vi "security system for building (2).vi"() -> ()   [LabVIEW 2020]
panel:
  out "Normal":bool
  out "Fire":bool
  in  "Temp":dbl
  in  "stop":bool
  out "Hot":bool
  out "Cold":bool
  in  "Switch":bool
  in  "Motion sensor":bool
  out "Light":bool
  in  "Stop Time":timestamp
  in  "Start Time":timestamp
  in  "ON/OFF":bool
  out "Normal Alarm":bool
  out "Smoke Alarm":bool
  out "Fire Alarm":bool
  in  "SMOKE LEVEL  SET POINT":dbl(knob) scale=0.0..100.0
  in  "SMOKE   DETECTOR":dbl(knob) scale=0.0..100.0
  in  "TEMP SET POINT":dbl(slide) scale=0.0..100.0
  in  "TEMPERATURE  DETECTOR":dbl(slide) scale=0.0..100.0
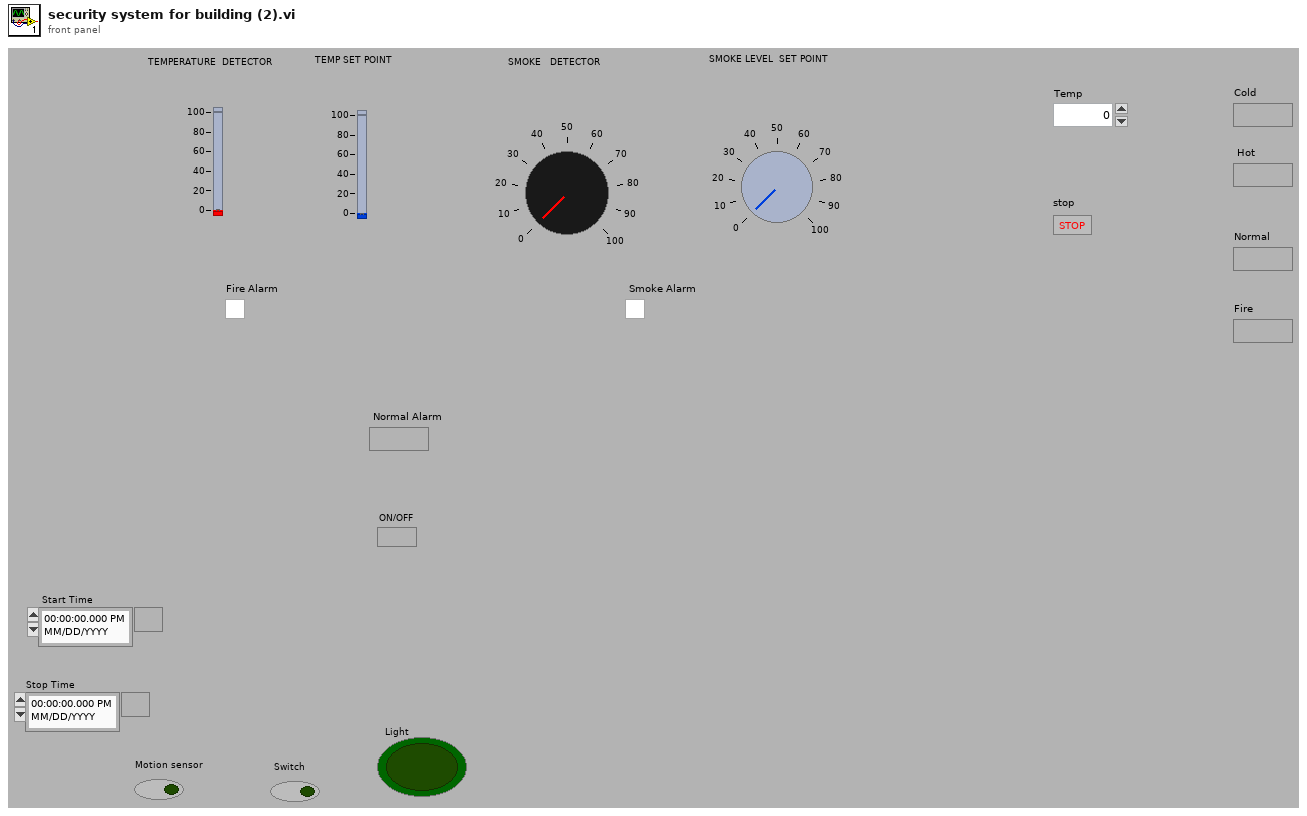
[diagram p1: front panel]
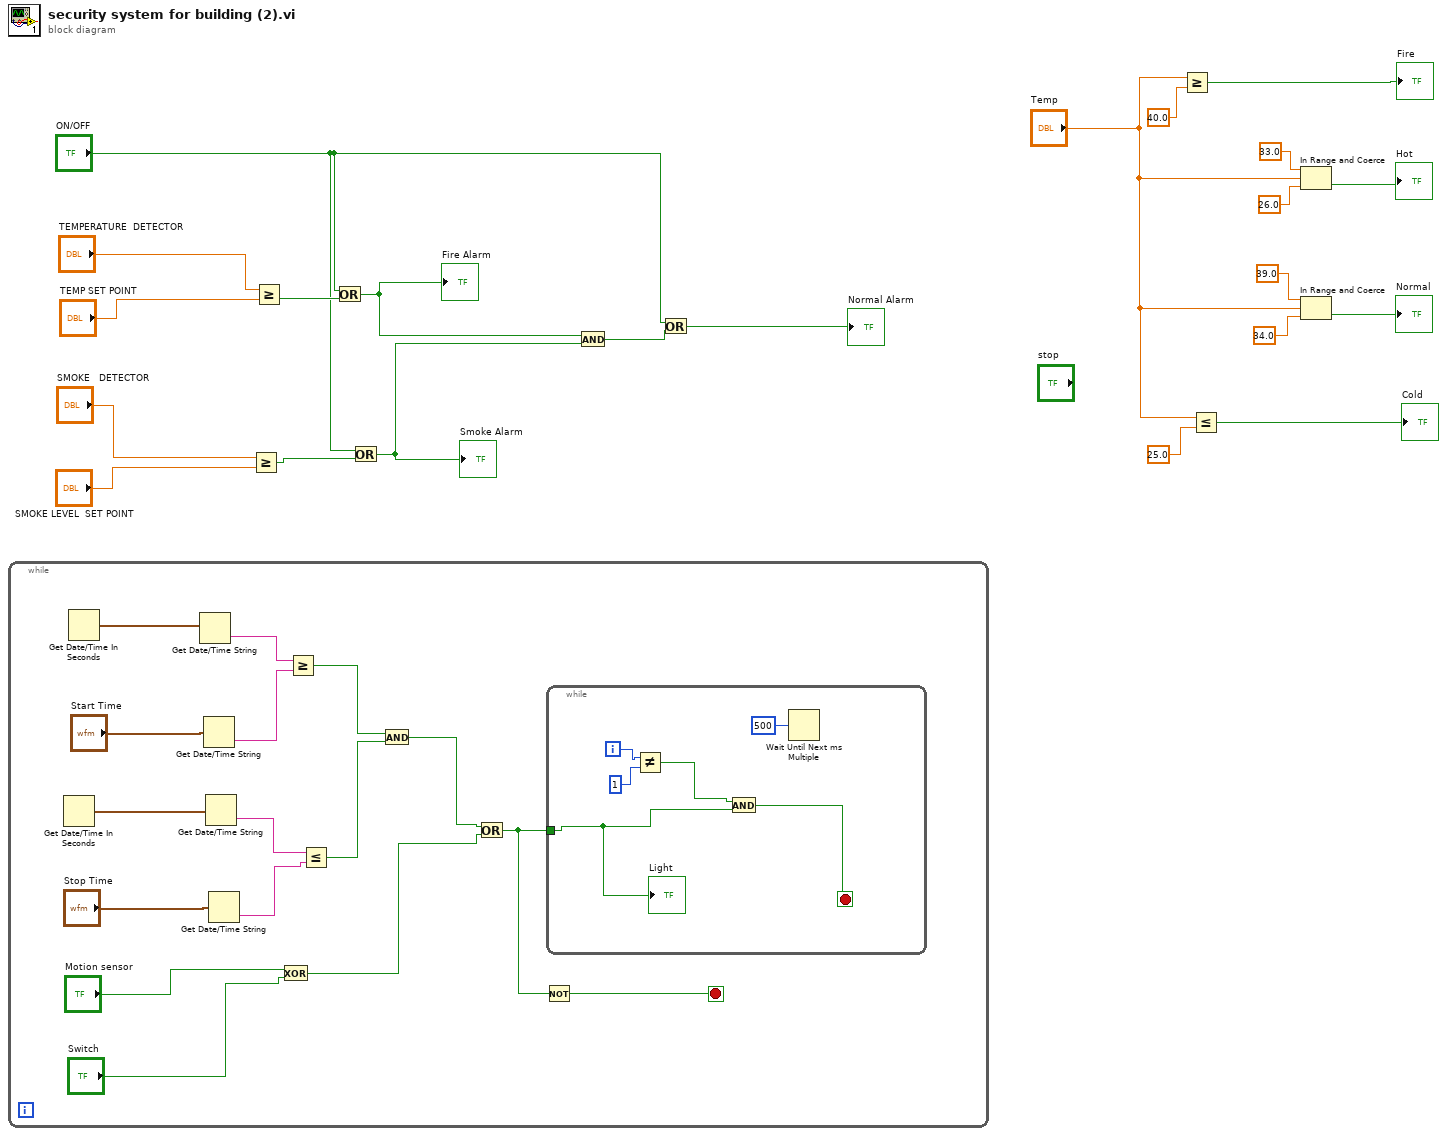
[diagram p0: block diagram]
diagram:
  n1 = while {
    stop <- w23 stop-if-true
    n2 = Get Date/Time In Seconds() -> (seconds since 1Jan1904=w36:timestamp)
    n3 = Get Date/Time In Seconds() -> (seconds since 1Jan1904=w38:timestamp)
    n4 = Get Date/Time String(seconds (now)=w38) -> (time string=w31:string)  [unwired: 2 in, 1 out]
    n5 = Get Date/Time String(seconds (now)="Start Time") -> (time string=w32:string)  [unwired: 2 in, 1 out]
    n6 = Get Date/Time String(seconds (now)=w36) -> (time string=w34:string)  [unwired: 2 in, 1 out]
    n7 = Get Date/Time String(seconds (now)="Stop Time") -> (time string=w33:string)  [unwired: 2 in, 1 out]
    n8 = Exclusive Or(1:"Switch", 2:"Motion sensor") -> (0:w25:bool)
    n9 = Greater Or Equal?(x=w31, y=w32) -> (x >= y?=w29:bool)
    n10 = Less Or Equal?(x=w34, y=w33) -> (x <= y?=w30:bool)
    n11 = And(x=w29, y=w30) -> (x .and. y?=w26:bool)
    n12 = Or(x=w26, y=w25) -> (x .or. y?=w24:bool)
    n13 = Not(x=w24) -> (.not. x?=w23:bool)
    n14 = while {
      tunnel: w24 -> [w42]
      i -> [w44]
      stop <- w40 stop-if-true
      n15 = Not Equal?(x=w44, y=1) -> (x != y?=w43:bool)
      n16 = And(x=w43, y=w42) -> (x .and. y?=w40:bool)
      n17 = Wait Until Next ms Multiple(millisecond multiple=500) -> ()  [unwired: 1 out]
      "Light" <- w42
    }
  }
  n18 = Greater Or Equal?(x="SMOKE   DETECTOR", y="SMOKE LEVEL  SET POINT") -> (x >= y?=w13:bool)
  n19 = Greater Or Equal?(x="TEMPERATURE  DETECTOR", y="TEMP SET POINT") -> (x >= y?=w18:bool)
  n20 = Or(x="ON/OFF", y=w18) -> (x .or. y?=w14:bool)
  "Fire Alarm" <- w14
  n21 = Or(x="ON/OFF", y=w13) -> (x .or. y?=w17:bool)
  "Smoke Alarm" <- w17
  n22 = And(x=w14, y=w17) -> (x .and. y?=w15:bool)
  n23 = Or(x="ON/OFF", y=w15) -> (x .or. y?=→"Normal Alarm":bool)
  n24 = Greater Or Equal?(x="Temp", y=40.0) -> (x >= y?=→"Fire":bool)
  n25 = Less Or Equal?(x="Temp", y=25.0) -> (x <= y?=→"Cold":bool)
  n26 = In Range and Coerce(upper limit=33.0, x="Temp", lower limit=26.0) -> (In Range?=→"Hot":bool)  [unwired: 1 out]
  n27 = In Range and Coerce(upper limit=39.0, x="Temp", lower limit=34.0) -> (In Range?=→"Normal":bool)  [unwired: 1 out]
